vi "C(T) global variables.vi"() -> ()   [LabVIEW 2016]
doc: "These are the \"executive\" global variables for the C(T) experiment\n\nPaul K Dixon\nPhysics 350\nCSUSB Physics"
panel:
  in  "error detect":bool
  in  "exec stop":bool
  # "C(T) Global variables"
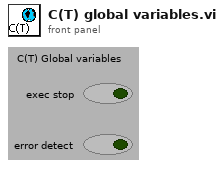
[diagram p1: front panel]
diagram:
